vi "isPath.vi"(7 "path Current VI":path, 8 "error in TCP":errorcluster, 10 "string Path in":string, 11 "connection ID in":refnum<k5>) -> (0 "error out TCP":errorcluster, 1 "Path is Ok?":bool, 2 "absolute path":path, 3 "connection ID out":refnum<k5>)   [LabVIEW 2010]
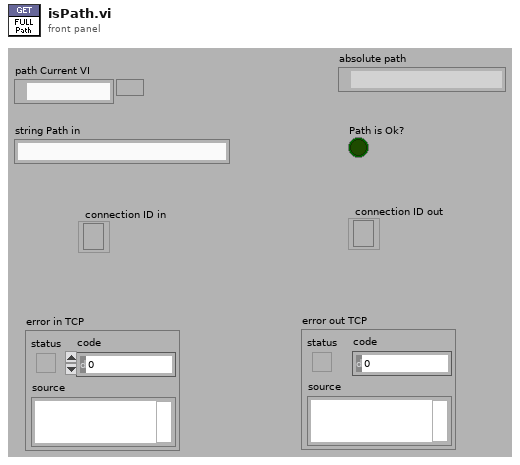
[diagram p1: front panel]
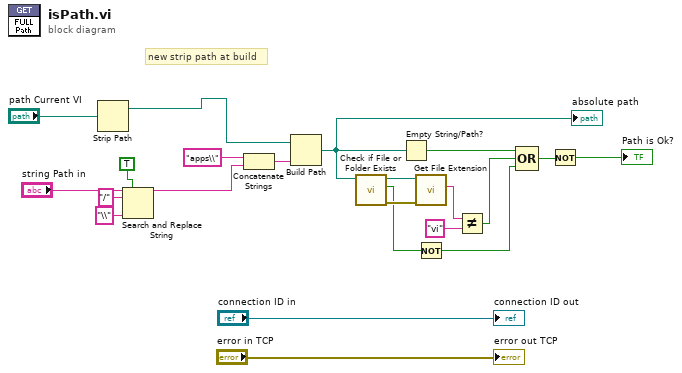
[diagram p0: block diagram]
diagram:
  # "new strip path at build"
  n1 = Strip Path(path="path Current VI") -> (stripped path=w1:path)  [unwired: 1 out]
  n2 = Search and Replace String(replace all?=TRUE ("replace all? (F)"), input string="string Path in", search string="/", replace string="\\" ("replace string (\"\")")) -> (result string=w5:string)  [unwired: 1 in, 6 out]
  n3 = Concatenate Strings("apps\\" ("string"), w5) -> (w22:string)
  n4 = Build Path(base path=w1, name or relative path=w22) -> (appended path=w13:path)
  "absolute path" <- w13
  n5 = call <vilib>:"Check if File or Folder Exists.vi"("path"=w13) -> ("error out"=w19:errorcluster, "file or folder exists?"=w15:bool, "dup path"=w20:path)  [unwired: 1 in, 7 out]
  n6 = Empty String/Path?(string/path=w13) -> (empty?=w17:bool)
  n7 = call <vilib>:"Get File Extension.vi"("error in (no error)"=w19, "file"=w20) -> ("lowercase file extension"=w2:string)  [unwired: 9 out]
  n8 = Not(x=w15) -> (.not. x?=w14:bool)
  n9 = Not Equal?(x=w2, y="vi") -> (x != y?=w16:bool)
  n10 = Compound Arithmetic op=OR(w17, w16, w14) -> (w4:bool)
  n11 = Not(x=w4) -> (.not. x?=→"Path is Ok?":bool)
  "connection ID out" <- "connection ID in"
  "error out TCP" <- "error in TCP"
